vi "autoGetIOData.vi"(11 "elapsed auton time":dbl) -> (3 "sensor datas":T2)   [LabVIEW 2013]
panel:
  out "output cluster":T1
  in  "const":T2
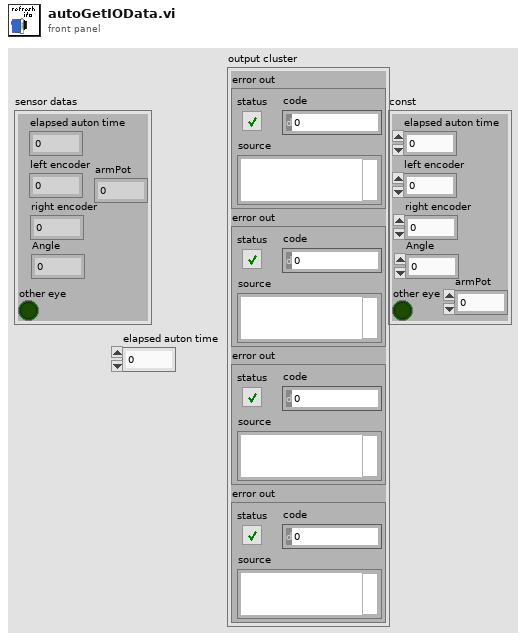
[diagram p1: front panel]
types:
  T1 = cluster{"error out":errorcluster, "error out":errorcluster, "error out":errorcluster, "error out":errorcluster}
  T2 = cluster{"elapsed auton time":dbl, "left encoder":dbl, "other eye":bool, "right encoder":dbl, "Angle":dbl, "armPot":dbl}
  T3 = typedef "WPI_GyroDevRef.ctl" = cluster{"DevStatus":errorcluster, "Analog Module":T4, "Analog Channel":T5, "Offset":dbl, "Gain (VoltsPerDegree/Second)":dbl}
  T4 = typedef "FPGA_TypedefAnalogModule.ctl" = enum16{"Analog Module 1", "Analog Module 2"}
  T5 = typedef "FPGA_AIChannel.ctl" = enum8{"AI 1", "AI 2", "AI 3", "AI 4", "AI 5", "AI 6", "AI 7", "AI 8", "Invalid"}
  T6 = typedef "WPI_EncoderDevRef.ctl" = cluster{"DevStatus":errorcluster, "EncoderIndex":T7, "CounterIndex":T8, "DistancePerCount":dbl, "Decoding Type":T9}
  T7 = typedef "FPGA_EncoderIdx.ctl" = enum8{"Enc 0", "Enc 1", "Enc 2", "Enc 3", "Invalid"}
  T8 = typedef "FPGA_CounterCtrSystemIndex.ctl" = enum8{"Ctr 0", "Ctr 1", "Ctr 2", "Ctr 3", "Ctr 4", "Ctr 5", "Ctr 6", "Ctr 7", "Invalid"}
  T9 = typedef "WPI_EncoderType.ctl" = enum16{"1x", "2x", "4x"}
  T10 = typedef "WPI_AnalogChannelDevRef.ctl" = cluster{"DevStatus":errorcluster, "Analog Module":T4, "Analog Channel":T5}
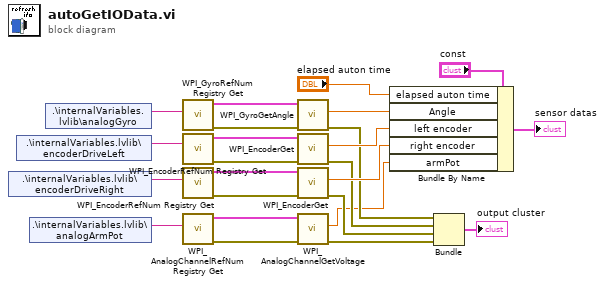
[diagram p0: block diagram]
diagram:
  n1 = shared-variable ".\\internalVariables.lvlib\\encoderDriveRight"() -> (w4:string)  [unwired: 1 in, 1 out]
  n2 = shared-variable ".\\internalVariables.lvlib\\encoderDriveLeft"() -> (w3:string)  [unwired: 1 in, 1 out]
  n3 = shared-variable ".\\internalVariables.lvlib\\analogArmPot"() -> (w5:string)  [unwired: 1 in, 1 out]
  n4 = shared-variable ".\\internalVariables.lvlib\\analogGyro"() -> (w2:string)  [unwired: 1 in, 1 out]
  n5 = call <vilib>:"WPI_GyroRefNum Registry Get.vi"("refnum name"=w2) -> ("error out"=w11:errorcluster, "GyroDevRef"=w12:T3)  [unwired: 9 in]
  n6 = call <vilib>:"WPI_EncoderRefNum Registry Get.vi"("refnum name"=w3) -> ("error out"=w15:errorcluster, "EncoderDevRef"=w16:T6)  [unwired: 9 in]
  n7 = call <vilib>:"WPI_EncoderRefNum Registry Get.vi"("refnum name"=w4) -> ("error out"=w14:errorcluster, "EncoderDevRef"=w13:T6)  [unwired: 9 in]
  n8 = call <vilib>:"WPI_AnalogChannelRefNum Registry Get.vi"("refnum name"=w5) -> ("error out"=w9:errorcluster, "AIDeviceRef"=w10:T10)  [unwired: 9 in]
  n9 = call <vilib>:"WPI_GyroGetAngle.vi"("error in (no error)"=w11, "GyroDevRef"=w12) -> ("error out"=w19:errorcluster, "Angle"=w22:dbl)  [unwired: 6 in, 2 out]
  n10 = call <vilib>:"WPI_EncoderGet.vi"("error in (no error)"=w15, "EncoderDevRef"=w16) -> ("error out"=w18:errorcluster, "Distance"=w21:dbl)  [unwired: 4 in, 4 out]
  n11 = call <vilib>:"WPI_EncoderGet.vi"("error in (no error)"=w14, "EncoderDevRef"=w13) -> ("error out"=w17:errorcluster, "Distance"=w20:dbl)  [unwired: 4 in, 4 out]
  n12 = call <vilib>:"WPI_AnalogChannelGetVoltage.vi"("error in (no error)"=w9, "AIDeviceRef"=w10) -> ("error out"=w8:errorcluster, "Voltage"=w1:dbl)  [unwired: 7 in, 1 out]
  n13 = Bundle By Name(cluster="const", "elapsed auton time"="elapsed auton time", "Angle"=w22, "left encoder"=w21, "right encoder"=w20, "armPot"=w1) -> (→"sensor datas":T2)
  n14 = Bundle("error out"=w19, "error out"=w18, "error out"=w17, "error out"=w8) -> (→"output cluster":T1)  [unwired: 1 in]
